vi "Begin.vi"() -> (0 "error out":errorcluster)   [LabVIEW 2013]
doc: "Called before other user functions, this VI is expected to open initial I/O refnums, load in file data, and do all program initialization. Notice that the <B>error out</B> terminal is simply used for data flow. Wiring it to other structures or subVIs ensures that this VI runs first."
uses:
  <vilib>/Rock Robotics/WPI/Camera/WPI_CameraImageSize.ctl
  <vilib>/Rock Robotics/SystemInterfaces/DIO/FPGA_DIOPWMChannel.ctl
  <vilib>/Rock Robotics/WPI/DriverStation/WPI_DriverStationRobotMode2.ctl
  <vilib>/Rock Robotics/WPI/Joystick/WPI_JoystickDeviceEnum.ctl
  <vilib>/Rock Robotics/SystemInterfaces/DIO/FPGA_DIOChannel.ctl
  <vilib>/Rock Robotics/WPI/Encoder/WPI_EncoderType.ctl
  <vilib>/Rock Robotics/WPI/Camera/WPI_CameraWhite Balance Values.ctl
  <vilib>/Rock Robotics/WPI/Camera/WPI_CameraExposure Values.ctl
  <vilib>/Rock Robotics/WPI/Camera/WPI_CameraFrameRate.ctl
  <vilib>/Rock Robotics/WPI/Solenoid/WPI_SolenoidChannel.ctl
  <vilib>/Rock Robotics/SystemInterfaces/DIO/FPGA_DIORelayChannel.ctl
  <vilib>/Rock Robotics/SystemInterfaces/Typedef/FPGA_TypedefDigitalModule.ctl
  <vilib>/Rock Robotics/SystemInterfaces/Typedef/FPGA_TypedefSolenoidModule.ctl
  <vilib>/Rock Robotics/SystemInterfaces/Typedef/FPGA_TypedefAnalogModule.ctl
  <vilib>/Rock Robotics/SystemInterfaces/AI/FPGA_AIChannel.ctl
  <vilib>/Rock Robotics/WPI/Relay/WPI_RelayDirection.ctl
  <vilib>/Rock Robotics/WPI/RobotDrive/WPI_RobotDriveOpen2MotorWithTalon.vi
  Robot Global Data.vi
  <vilib>/Rock Robotics/WPI/MotorControl/WPI_MotorControlOpen Talon.vi
  <vilib>/Rock Robotics/WPI/Counter/WPI_CounterDigitalInputToDigitalSource.vi
  <vilib>/Rock Robotics/WPI/Solenoid/WPI_SolenoidOpenDouble.vi
  <vilib>/Rock Robotics/WPI/Compressor/WPI_CompressorGetSetRefNum.vi
panel:
  in  "Image Size 2":T1=enum."160x120"
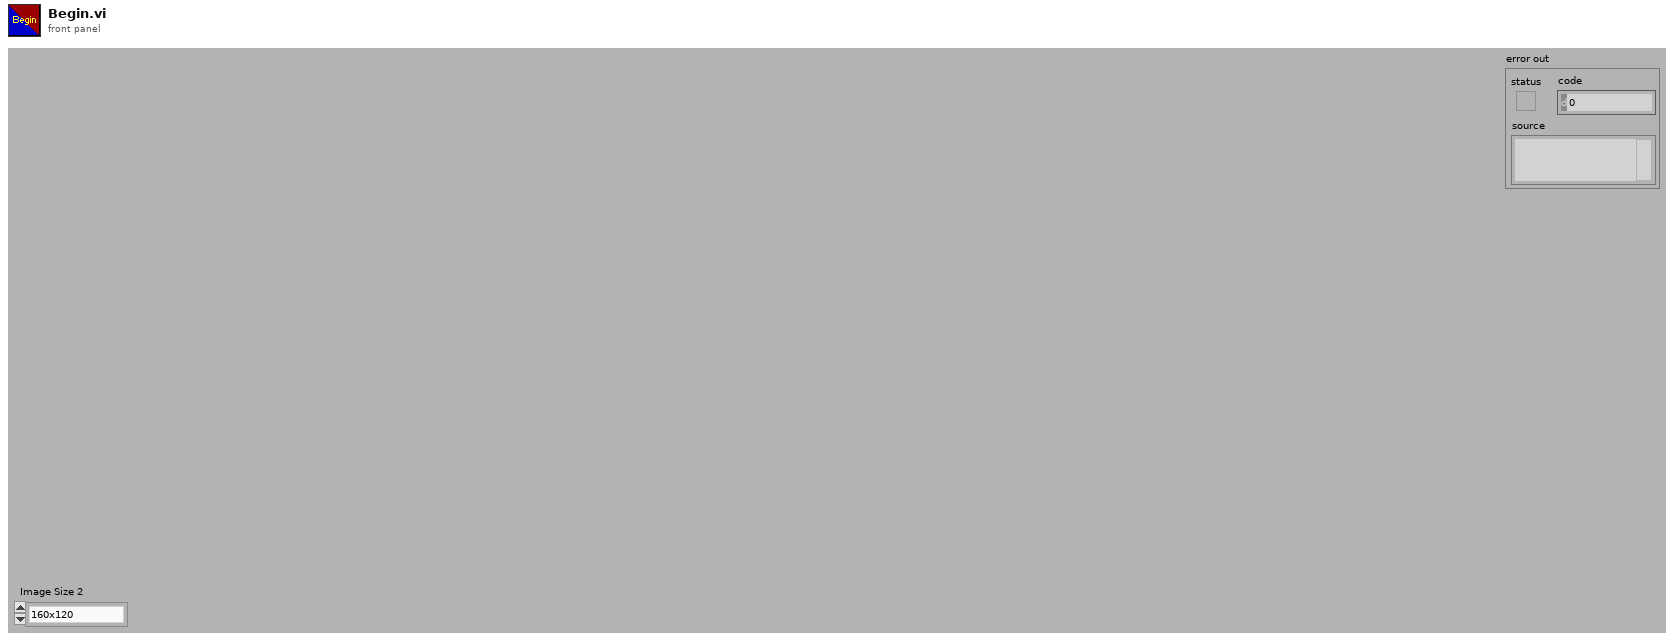
[diagram p1: front panel]
types:
  T1 = typedef "WPI_CameraImageSize.ctl" = enum16{"640x480", "320x240", "160x120"}
  T2 = typedef "WPI_RelayDirection.ctl" = enum16{"Both directions", "Forward only", "Reverse only"}
  T3 = typedef "FPGA_DIORelayChannel.ctl" = enum8{"Relay 1", "Relay 2", "Relay 3", "Relay 4", "Relay 5", "Relay 6", "Relay 7", "Relay 8", "Invalid"}
  T4 = typedef "FPGA_TypedefDigitalModule.ctl" = enum16{"Digital Module 1", "Digital Module 2"}
  T5 = typedef "FPGA_DIOChannel.ctl" = enum8{"DIO 1", "DIO 2", "DIO 3", "DIO 4", "DIO 5", "DIO 6", "DIO 7", "DIO 8", "DIO 9", "DIO 10", "DIO 11", "DIO 12", "DIO 13", "DIO 14", "Invalid"}
  T6 = typedef "WPI_EncoderType.ctl" = enum16{"1x", "2x", "4x"}
  T7 = typedef "FPGA_AIChannel.ctl" = enum8{"AI 1", "AI 2", "AI 3", "AI 4", "AI 5", "AI 6", "AI 7", "AI 8", "Invalid"}
  T8 = typedef "FPGA_TypedefAnalogModule.ctl" = enum16{"Analog Module 1", "Analog Module 2"}
  T9 = typedef "WPI_SolenoidChannel.ctl" = enum8{"Solenoid 1", "Solenoid 2", "Solenoid 3", "Solenoid 4", "Solenoid 5", "Solenoid 6", "Solenoid 7", "Solenoid 8", "Invalid"}
  T10 = typedef "FPGA_TypedefSolenoidModule.ctl" = enum16{"Solenoid Module 1", "Solenoid Module 2"}
  T11 = typedef "FPGA_DIOPWMChannel.ctl" = enum8{"PWM 1", "PWM 2", "PWM 3", "PWM 4", "PWM 5", "PWM 6", "PWM 7", "PWM 8", "PWM 9", "PWM 10", "Invalid"}
  T12 = typedef "WPI_CameraFrameRate.ctl" = u32
  T13 = typedef "WPI_CameraExposure Values.ctl" = enum16{"Auto", "Flicker-free 50 Hz", "Flicker-free 60 Hz", "Hold current"}
  T14 = typedef "WPI_CameraWhite Balance Values.ctl" = enum16{"Auto", "Fixed indoor", "Fixed outdoor 1", "Fixed outdoor 2", "Fixed fluorescent 1", "Fixed fluorescent 2", "Hold current"}
  T15 = typedef "WPI_JoystickDeviceEnum.ctl" = enum16{"USB 1", "USB 2", "USB 3", "USB 4", "Kinect 1", "Kinect 2"}
  T16 = typedef "WPI_DriverStationRobotMode2.ctl" = enum16{"Autonomous Disabled", "Autonomous Enabled", "Teleop Disabled", "Teleop Enabled", "Timeout", "Finish", "Test Disabled", "Test Enabled"}
  T17 = typedef "WPI_JoystickDevRef.ctl" = cluster{"Device":T15}
  T18 = typedef "WPI_DigitalInputDevRef.ctl" = cluster{"DevStatus":errorcluster, "DIO Channel":T5, "Digital Module":T4}
  T19 = typedef "WPI_CompressorDevRef.ctl" = cluster{"DevStatus":errorcluster, "DigitalInputDevRef":T18, "RelayDevRef":T20}
  T20 = typedef "WPI_RelayDevRef.ctl" = cluster{"DevStatus":errorcluster, "Relay Channel":T3, "Digital Module":T4, "Relay Direction":T2}
  T21 = typedef "WPI_RobotDriveDevRef.ctl" = cluster{"DevStatus":errorcluster, "Motors[]":T22[], "Square Inputs":bool, "Max Output":dbl, "Isochronous":bool}
  T22 = typedef "WPI_MotorControlDeviceRef.ctl" = cluster{"DeviceStatus":errorcluster, "Type":enum16{"PWM", "CAN"}, "PWM":cluster{"Digital Module":T4, "PWM Channel":T11, "DeadBand":T23}, "CAN":cluster{"Device Number":u8, "Control Mode":T24, "Semaphore":T25, "Max Vout":dbl}, "Invert":bool, "TransformRef":T26, "InvTransformRef":T26}
  T23 = typedef "WPI_PWMDeadband.ctl" = cluster{"Name":string, "maxPositivePwm":i32, "minPositivePwm":i32, "centerPwm":i32, "maxNegativePwm":i32, "minNegativePwm":i32, "angularRange":u16}
  T24 = typedef "WPI_CANJaguar_ControlMode.ctl" = enum8{"Percent VBus", "Current", "Speed", "Position", "Voltage"}
  T25 = typedef "Semaphore RefNum" = refnum<k1>
  T26 = typedef "WPI_PWMTransform_ConPane.ctl" = refnum<vi>
  T27 = typedef "WPI_SolenoidDevRef.ctl" = cluster{"DevStatus":errorcluster, "Solenoid Module":T10, "Forward Solenoid Channel":T9, "Reverse Solenoid Channel":T9}
  T28 = typedef "FPGA_CounterEncoderSourceConvertionLVSourceType.ctl" = cluster{"DevStatus":errorcluster, "AnalogTriggerMode?":bool, "DigitalMode":cluster{"Digital Module":T4, "DIO Channel":T29}, "AnalogTriggerMode":cluster{"AnalogTriggerIndex":T30, "OutputType":T31}}
  T29 = typedef "FPGA_DIODigitalSourceChannel.ctl" = enum8{"DIO 1", "DIO 2", "DIO 3", "DIO 4", "DIO 5", "DIO 6", "DIO 7", "DIO 8", "DIO 9", "DIO 10", "DIO 11", "DIO 12", "DIO 13", "DIO 14", "Disabled"}
  T30 = typedef "FPGA_AnalogTriggerIndex.ctl" = enum8{"Trig 0", "Trig 1", "Trig 2", "Trig 3", "Trig 4", "Trig 5", "Trig 6", "Trig 7", "Invalid"}
  T31 = typedef "FPGA_AnalogTriggerOutType.ctl" = enum16{"InWindow", "TriggerState", "Rising", "Falling"}
  T32 = typedef "WPI_EncoderDevRef.ctl" = cluster{"DevStatus":errorcluster, "EncoderIndex":T33, "CounterIndex":T34, "DistancePerCount":dbl, "Decoding Type":T6}
  T33 = typedef "FPGA_EncoderIdx.ctl" = enum8{"Enc 0", "Enc 1", "Enc 2", "Enc 3", "Invalid"}
  T34 = typedef "FPGA_CounterCtrSystemIndex.ctl" = enum8{"Ctr 0", "Ctr 1", "Ctr 2", "Ctr 3", "Ctr 4", "Ctr 5", "Ctr 6", "Ctr 7", "Invalid"}
  T35 = typedef "WPI_CameraDevRef.ctl" = cluster{"Camera Address":string, "CameraStatus":errorcluster, "Acquire Image Notifier":refnum<notifier>}
  T36 = typedef "WPI_ServoDeviceRef.ctl" = cluster{"DeviceStatus":errorcluster, "Digital Module":T4, "PWM Channel":T11, "DeadBand":T23}
  T37 = typedef "WPI_AnalogChannelDevRef.ctl" = cluster{"DevStatus":errorcluster, "Analog Module":T8, "Analog Channel":T7}
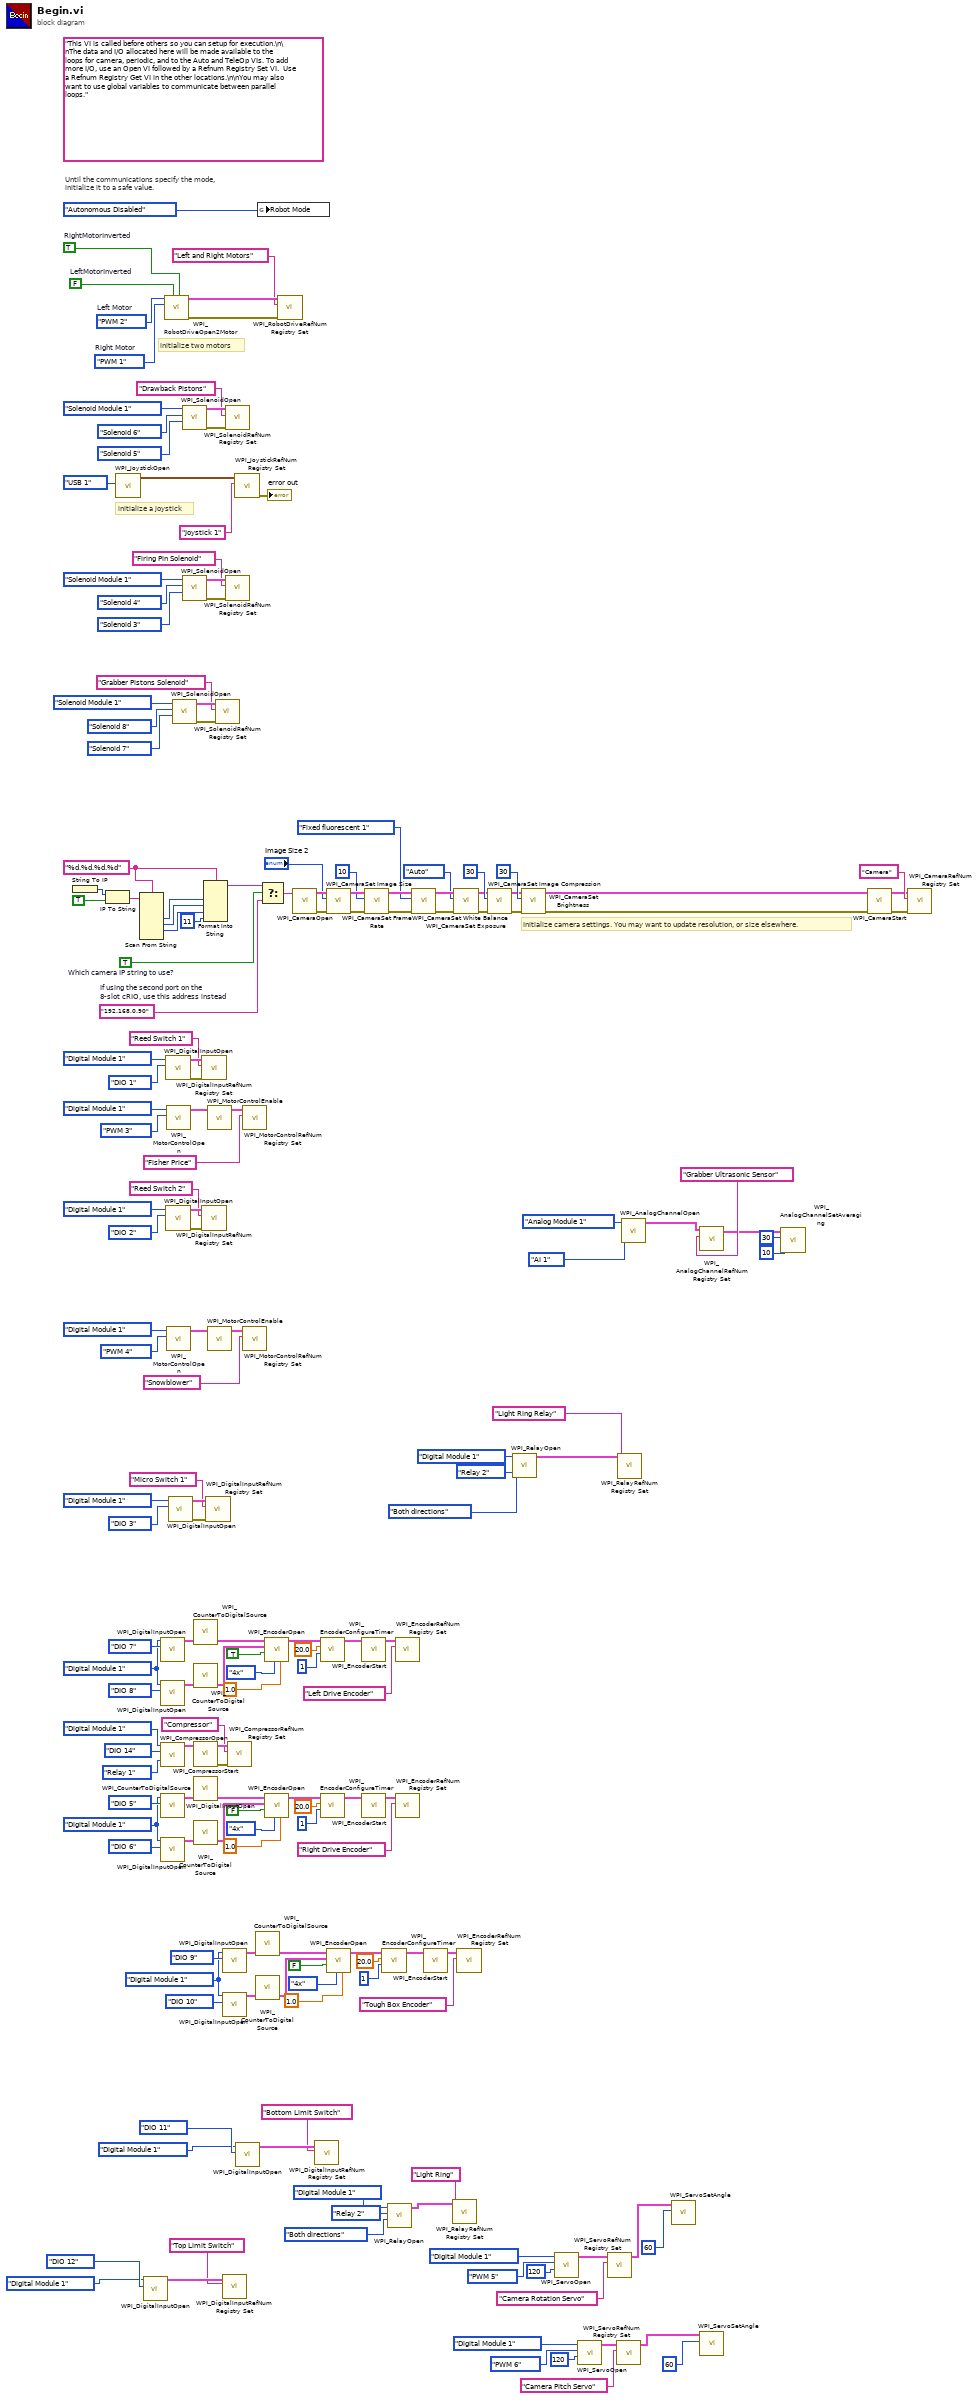
[diagram p0: block diagram]
diagram:
  w22 = FPGA_TypedefDigitalModule."Digital Module 1" ("DIO Module")
  w69 = FPGA_TypedefDigitalModule."Digital Module 1" ("DIO Module")
  w121 = TRUE  # Which camera IP string to use?
  w125 = "%d.%d.%d.%d" ("format string")
  w122 = "192.168.0.90"  # If using the second port on the 8-slot cRIO, use this address instead
  w154 = FPGA_TypedefDigitalModule."Digital Module 1" ("DIO Module")
  (unwired) "This VI is called before others so you can setup for execution.\n\nThe data and I/O allocated here will be made available to the loops for camera, periodic, and to the Auto and TeleOp VIs. To add more I/O, use an Open VI followed by a Refnum Registry Set VI.  Use a Refnum Registry Get VI in the other locations.\n\nYou may also want to use global variables to communicate between parallel loops."
  w178 = FPGA_DIOPWMChannel."PWM 1"  # Right Motor
  w179 = FPGA_DIOPWMChannel."PWM 2"  # Left Motor
  w183 = FALSE  # LeftMotorInverted
  w184 = TRUE  # RightMotorInverted
  # "Initialize camera settings. You may want to update resolution, or size elsewhere."
  # "initialize a joystick"
  # "Until the communications specify the mode,\ninitialize it to a safe value."
  # "initialize two motors"
  n1 = String To IP() -> (0:w132:u32)  [unwired: 1 in]
  n2 = IP To String(1:TRUE ("dot notation? (F)"), 2:w132) -> (0:w130:string)
  n3 = call <vilib>:"WPI_JoystickOpen.vi"("JoystickDevice"=WPI_JoystickDeviceEnum."USB 1") -> ("JoystickDevRef"=w175:T17)  [unwired: 10 in]
  n4 = Scan From String(format string=w125, input string=w130) -> (output 1=w129:i32, output 2=w128:i32, output 3=w127:i32)  [unwired: 7 in, 3 out]
  n5 = call <vilib>:"WPI_DigitalInputOpen.vi"("DIO Channel"=FPGA_DIOChannel."DIO 12" ("A Channel"), "Digital Module (Module 1)"=FPGA_TypedefDigitalModule."Digital Module 1" ("DIO Module")) -> ("DigitalInputDevRef"=w37:T18)  [unwired: 8 in, 1 out]
  n6 = call <vilib>:"WPI_DigitalInputOpen.vi"("DIO Channel"=FPGA_DIOChannel."DIO 7" ("A Channel"), "Digital Module (Module 1)"=w22) -> ("DigitalInputDevRef"=w33:T18)  [unwired: 1 in, 8 out]
  n7 = call <vilib>:"WPI_DigitalInputOpen.vi"("DIO Channel"=FPGA_DIOChannel."DIO 8" ("B Channel"), "Digital Module (Module 1)"=w22) -> ("DigitalInputDevRef"=w34:T18)  [unwired: 1 in, 8 out]
  n8 = call <vilib>:"WPI_CompressorOpen.vi"("Pressure Switch Digital Module (Module 1)"=FPGA_TypedefDigitalModule."Digital Module 1" ("Switch and Relay Module"), "Pressure Switch DIO Channel"=FPGA_DIOChannel."DIO 14" ("Pressure Switch Channel"), "Relay Channel"=FPGA_DIORelayChannel."Relay 1" ("RelayChannel")) -> ("CompressorDevRef"=w109:T19)  [unwired: 2 in, 10 out]
  n9 = call <vilib>:"WPI_DigitalInputOpen.vi"("DIO Channel"=FPGA_DIOChannel."DIO 5" ("A Channel"), "Digital Module (Module 1)"=w154) -> ("DigitalInputDevRef"=w165:T18)  [unwired: 1 in, 8 out]
  n10 = call <vilib>:"WPI_DigitalInputOpen.vi"("DIO Channel"=FPGA_DIOChannel."DIO 6" ("B Channel"), "Digital Module (Module 1)"=w154) -> ("DigitalInputDevRef"=w166:T18)  [unwired: 1 in, 8 out]
  n11 = call-poly <vilib>:"WPI_RobotDriveOpen2Motor.vi"("Right Motor Inverted"=w184, "Left Motor Inverted"=w183, "Right Motor"=w178, "Left Motor"=w179) -> ("error out"=w180:errorcluster, "RobotDriveDevRef"=w182:T21)  [unwired: 1 in, 5 out]
  n12 = call <vilib>:"WPI_DigitalInputOpen.vi"("DIO Channel"=FPGA_DIOChannel."DIO 1" ("Limit Switch Channel"), "Digital Module (Module 1)"=FPGA_TypedefDigitalModule."Digital Module 1" ("Switch and Relay Module")) -> ("error out"=w108:errorcluster, "DigitalInputDevRef"=w107:T18)  [unwired: 1 in, 7 out]
  n13 = call <vilib>:"WPI_DigitalInputOpen.vi"("DIO Channel"=FPGA_DIOChannel."DIO 2" ("Limit Switch Channel"), "Digital Module (Module 1)"=FPGA_TypedefDigitalModule."Digital Module 1" ("Switch and Relay Module")) -> ("error out"=w90:errorcluster, "DigitalInputDevRef"=w89:T18)  [unwired: 1 in, 7 out]
  n14 = call-poly <vilib>:"WPI_MotorControlOpen.vi"("PWM Channel"=FPGA_DIOPWMChannel."PWM 3" ("Left Motor"), "Digital Module (Module 1)"=enum16{"Digital Module 1"}."Digital Module 1") -> ("MotorControlDeviceRef"=w86:T22)  [unwired: 8 in, 1 out]
  n15 = call-poly <vilib>:"WPI_MotorControlOpen.vi"("PWM Channel"=FPGA_DIOPWMChannel."PWM 4" ("Left Motor"), "Digital Module (Module 1)"=enum16{"Digital Module 1"}."Digital Module 1") -> ("MotorControlDeviceRef"=w84:T22)  [unwired: 8 in, 1 out]
  n16 = call <vilib>:"WPI_DigitalInputOpen.vi"("DIO Channel"=FPGA_DIOChannel."DIO 3", "Digital Module (Module 1)"=FPGA_TypedefDigitalModule."Digital Module 1") -> ("error out"=w16:errorcluster, "DigitalInputDevRef"=w17:T18)  [unwired: 1 in, 7 out]
  n17 = call-poly <vilib>:"WPI_SolenoidOpen.vi"("Reverse Solenoid Channel"=WPI_SolenoidChannel."Solenoid 7" ("Extend Solenoid Channel"), "Forward Solenoid Channel"=WPI_SolenoidChannel."Solenoid 8" ("Retract Solenoid Channel"), "Solenoid Module (Module 1)"=FPGA_TypedefSolenoidModule."Solenoid Module 1" ("Solenoid Module")) -> ("error out"=w49:errorcluster, "SolenoidDevRef"=w48:T27)  [unwired: 1 in, 6 out]
  n18 = call-poly <vilib>:"WPI_SolenoidOpen.vi"("Reverse Solenoid Channel"=WPI_SolenoidChannel."Solenoid 5" ("Extend Solenoid Channel"), "Forward Solenoid Channel"=WPI_SolenoidChannel."Solenoid 6" ("Retract Solenoid Channel"), "Solenoid Module (Module 1)"=FPGA_TypedefSolenoidModule."Solenoid Module 1" ("Solenoid Module")) -> ("error out"=w105:errorcluster, "SolenoidDevRef"=w104:T27)  [unwired: 1 in, 6 out]
  n19 = call-poly <vilib>:"WPI_SolenoidOpen.vi"("Reverse Solenoid Channel"=WPI_SolenoidChannel."Solenoid 3" ("Extend Solenoid Channel"), "Forward Solenoid Channel"=WPI_SolenoidChannel."Solenoid 4" ("Retract Solenoid Channel"), "Solenoid Module (Module 1)"=FPGA_TypedefSolenoidModule."Solenoid Module 1" ("Solenoid Module")) -> ("error out"=w96:errorcluster, "SolenoidDevRef"=w95:T27)  [unwired: 1 in, 6 out]
  n20 = call-poly <vilib>:"WPI_CounterToDigitalSource.vi"("DigitalInputDevRef"=w33) -> ("Digital Source"=w32:T28)  [unwired: 6 out]
  n21 = call-poly <vilib>:"WPI_CounterToDigitalSource.vi"("DigitalInputDevRef"=w34) -> ("Digital Source"=w35:T28)  [unwired: 6 out]
  n22 = call <vilib>:"WPI_CompressorStart.vi"("CompressorDevRef"=w109) -> ("error out"=w102:errorcluster, "CompressorDevRef"=w101:T19)  [unwired: 1 in, 8 out]
  n23 = call-poly <vilib>:"WPI_CounterToDigitalSource.vi"("DigitalInputDevRef"=w165) -> ("Digital Source"=w164:T28)  [unwired: 6 out]
  n24 = call-poly <vilib>:"WPI_CounterToDigitalSource.vi"("DigitalInputDevRef"=w166) -> ("Digital Source"=w167:T28)  [unwired: 6 out]
  n25 = call <vilib>:"WPI_DigitalInputRefNum Registry Set.vi"("error in (no error)"=w108, "refnum name"="Reed Switch 1", "DigitalInputDevRef"=w107) -> ()  [unwired: 7 in, 2 out]
  n26 = call <vilib>:"WPI_DigitalInputRefNum Registry Set.vi"("error in (no error)"=w90, "refnum name"="Reed Switch 2", "DigitalInputDevRef"=w89) -> ()  [unwired: 7 in, 2 out]
  n27 = Format Into String(format string=w125, w129, w128, w127, 11 ("Compression")) -> (resulting string=w123:string)  [unwired: 2 in, 1 out]
  n28 = call <vilib>:"WPI_DigitalInputRefNum Registry Set.vi"("error in (no error)"=w16, "refnum name"="Micro Switch 1", "DigitalInputDevRef"=w17) -> ()  [unwired: 7 in, 2 out]
  n29 = call <vilib>:"WPI_MotorControlEnable.vi"("CAN Jaguar Ref"=w86) -> ("CAN Jaguar Ref Out"=w85:T22)  [unwired: 9 in, 1 out]
  n30 = call <vilib>:"WPI_MotorControlEnable.vi"("CAN Jaguar Ref"=w84) -> ("CAN Jaguar Ref Out"=w83:T22)  [unwired: 9 in, 1 out]
  n31 = call <vilib>:"WPI_SolenoidRefNum Registry Set.vi"("error in (no error)"=w49, "refnum name"="Grabber Pistons Solenoid", "SolenoidDevRef"=w48) -> ()  [unwired: 7 in, 2 out]
  n32 = call <vilib>:"WPI_DigitalInputOpen.vi"("DIO Channel"=FPGA_DIOChannel."DIO 9" ("A Channel"), "Digital Module (Module 1)"=w69) -> ("DigitalInputDevRef"=w80:T18)  [unwired: 1 in, 8 out]
  n33 = call <vilib>:"WPI_DigitalInputOpen.vi"("DIO Channel"=FPGA_DIOChannel."DIO 10" ("B Channel"), "Digital Module (Module 1)"=w69) -> ("DigitalInputDevRef"=w81:T18)  [unwired: 1 in, 8 out]
  n34 = call <vilib>:"WPI_DigitalInputRefNum Registry Set.vi"("refnum name"="Top Limit Switch", "DigitalInputDevRef"=w37) -> ()  [unwired: 8 in, 2 out]
  n35 = call <vilib>:"WPI_SolenoidRefNum Registry Set.vi"("error in (no error)"=w105, "refnum name"="Drawback Pistons", "SolenoidDevRef"=w104) -> ()  [unwired: 7 in, 2 out]
  n36 = call <vilib>:"WPI_SolenoidRefNum Registry Set.vi"("error in (no error)"=w96, "refnum name"="Firing Pin Solenoid", "SolenoidDevRef"=w95) -> ()  [unwired: 7 in, 2 out]
  n37 = call <vilib>:"WPI_CompressorRefNum Registry Set.vi"("error in (no error)"=w102, "refnum name"="Compressor", "CompressorDevRef"=w101) -> ()  [unwired: 7 in, 2 out]
  n38 = call <vilib>:"WPI_JoystickRefNum Registry Set.vi"("refnum name"="Joystick 1", "JoystickDevRef"=w175) -> ("error out"=→"error out":errorcluster)  [unwired: 8 in, 1 out]
  n39 = call <vilib>:"WPI_DigitalInputOpen.vi"("DIO Channel"=FPGA_DIOChannel."DIO 11" ("A Channel"), "Digital Module (Module 1)"=FPGA_TypedefDigitalModule."Digital Module 1" ("DIO Module")) -> ("DigitalInputDevRef"=w64:T18)  [unwired: 8 in, 1 out]
  n40 = call <vilib>:"WPI_MotorControlRefNum Registry Set.vi"("refnum name"="Fisher Price", "MotorControlDevRef"=w85) -> ()  [unwired: 8 in, 2 out]
  n41 = call <vilib>:"WPI_MotorControlRefNum Registry Set.vi"("refnum name"="Snowblower", "MotorControlDevRef"=w83) -> ()  [unwired: 8 in, 2 out]
  n42 = call-poly <vilib>:"WPI_CounterToDigitalSource.vi"("DigitalInputDevRef"=w80) -> ("Digital Source"=w79:T28)  [unwired: 6 out]
  n43 = call-poly <vilib>:"WPI_CounterToDigitalSource.vi"("DigitalInputDevRef"=w81) -> ("Digital Source"=w82:T28)  [unwired: 6 out]
  n44 = global write "Robot Global Data.vi" "Robot Mode"(WPI_DriverStationRobotMode2."Autonomous Disabled" ("Robot Mode")) -> ()
  n45 = Select(t=w123, s=w121, f=w122) -> (s? t:f=w124:string)
  n46 = call <vilib>:"WPI_EncoderOpen.vi"("DistancePerCount"=1.0, "Decoding Type"=WPI_EncoderType."4x", "Invert Direction (False)"=TRUE ("Invert Direction"), "BSource"=w35, "ASource"=w32) -> ("EncoderDevRef"=w25:T32)  [unwired: 3 in, 3 out]
  n47 = call <vilib>:"WPI_EncoderOpen.vi"("DistancePerCount"=1.0, "Decoding Type"=WPI_EncoderType."4x", "Invert Direction (False)"=FALSE ("Invert Direction"), "BSource"=w167, "ASource"=w164) -> ("EncoderDevRef"=w157:T32)  [unwired: 3 in, 3 out]
  n48 = call <vilib>:"WPI_RobotDriveRefNum Registry Set.vi"("error in (no error)"=w180, "refnum name"="Left and Right Motors", "RobotDriveDevRef"=w182) -> ()  [unwired: 9 out]
  n49 = call <vilib>:"WPI_CameraOpen.vi"("Camera Address"=w124) -> ("error out"=w142:errorcluster, "CameraDevRef"=w143:T35)  [unwired: 1 in, 8 out]
  n50 = call <vilib>:"WPI_DigitalInputRefNum Registry Set.vi"("refnum name"="Bottom Limit Switch", "DigitalInputDevRef"=w64) -> ()  [unwired: 8 in, 2 out]
  n51 = call <vilib>:"WPI_EncoderConfigureTimer.vi"("Number Samples to Average"=u8 1, "Minimum Rate"=20.0, "EncoderDevRef"=w25) -> ("EncoderDevRef"=w26:T32)  [unwired: 1 in, 7 out]
  n52 = call <vilib>:"WPI_EncoderConfigureTimer.vi"("Number Samples to Average"=u8 1, "Minimum Rate"=20.0, "EncoderDevRef"=w157) -> ("EncoderDevRef"=w158:T32)  [unwired: 1 in, 7 out]
  n53 = call <vilib>:"WPI_CameraSet Image Size.vi"("error in (no error)"=w142, "Image Size"="Image Size 2", "CameraDevRef"=w143) -> ("error out"=w141:errorcluster, "CameraDevRef Out"=w144:T35)  [unwired: 7 out]
  n54 = call <vilib>:"WPI_EncoderOpen.vi"("DistancePerCount"=1.0, "Decoding Type"=WPI_EncoderType."4x", "Invert Direction (False)"=FALSE ("Invert Direction"), "BSource"=w82, "ASource"=w79) -> ("EncoderDevRef"=w72:T32)  [unwired: 3 in, 3 out]
  n55 = call <vilib>:"WPI_EncoderStart.vi"("EncoderDevRef"=w26) -> ("EncoderDevRef"=w21:T32)  [unwired: 1 in, 9 out]
  n56 = call <vilib>:"WPI_EncoderStart.vi"("EncoderDevRef"=w158) -> ("EncoderDevRef"=w153:T32)  [unwired: 1 in, 9 out]
  n57 = call <vilib>:"WPI_CameraSet Frame Rate.vi"("error in (no error)"=w141, "Frame Rate (fps)"=T12 10, "CameraDevRef"=w144) -> ("error out"=w140:errorcluster, "CameraDevRef Out"=w146:T35)  [unwired: 7 out]
  n58 = call <vilib>:"WPI_EncoderConfigureTimer.vi"("Number Samples to Average"=u8 1, "Minimum Rate"=20.0, "EncoderDevRef"=w72) -> ("EncoderDevRef"=w73:T32)  [unwired: 1 in, 7 out]
  n59 = call <vilib>:"WPI_RelayOpen.vi"("Relay Direction"=WPI_RelayDirection."Both directions", "Relay Channel"=FPGA_DIORelayChannel."Relay 2", "Digital Module (Module 1)"=FPGA_TypedefDigitalModule."Digital Module 1") -> ("RelayDevRef"=w6:T20)  [unwired: 7 in, 1 out]
  n60 = call <vilib>:"WPI_EncoderRefNum Registry Set.vi"("refnum name"="Left Drive Encoder", "EncoderDevRef"=w21) -> ()  [unwired: 8 in, 2 out]
  n61 = call <vilib>:"WPI_EncoderRefNum Registry Set.vi"("refnum name"="Right Drive Encoder", "EncoderDevRef"=w153) -> ()  [unwired: 8 in, 2 out]
  n62 = call <vilib>:"WPI_CameraSet White Balance.vi"("error in (no error)"=w140, "White Balance"=WPI_CameraWhite_Balance_Values."Fixed fluorescent 1", "CameraDevRef"=w146) -> ("error out"=w139:errorcluster, "CameraDevRef Out"=w145:T35)  [unwired: 7 out]
  n63 = call <vilib>:"WPI_EncoderStart.vi"("EncoderDevRef"=w73) -> ("EncoderDevRef"=w68:T32)  [unwired: 1 in, 9 out]
  n64 = call <vilib>:"WPI_RelayRefNum Registry Set.vi"("refnum name"="Light Ring", "RelayDevRef"=w6) -> ()  [unwired: 8 in, 2 out]
  n65 = call <vilib>:"WPI_CameraSet Exposure.vi"("error in (no error)"=w139, "Exposure"=WPI_CameraExposure_Values."Auto", "CameraDevRef"=w145) -> ("error out"=w138:errorcluster, "CameraDevRef Out"=w148:T35)  [unwired: 7 out]
  n66 = call <vilib>:"WPI_EncoderRefNum Registry Set.vi"("refnum name"="Tough Box Encoder", "EncoderDevRef"=w68) -> ()  [unwired: 8 in, 2 out]
  n67 = call <vilib>:"WPI_CameraSet Image Compression.vi"("error in (no error)"=w138, "Compression"=30, "CameraDevRef"=w148) -> ("error out"=w137:errorcluster, "CameraDevRef Out"=w147:T35)  [unwired: 7 out]
  n68 = call <vilib>:"WPI_RelayOpen.vi"("Relay Direction"=WPI_RelayDirection."Both directions", "Relay Channel"=FPGA_DIORelayChannel."Relay 2", "Digital Module (Module 1)"=FPGA_TypedefDigitalModule."Digital Module 1") -> ("RelayDevRef"=w11:T20)  [unwired: 7 in, 1 out]
  n69 = call <vilib>:"WPI_CameraSet Brightness.vi"("error in (no error)"=w137, "Brightness"=30, "CameraDevRef"=w147) -> ("error out"=w120:errorcluster, "CameraDevRef Out"=w119:T35)  [unwired: 7 out]
  n70 = call <vilib>:"WPI_ServoOpen.vi"("Angular Range"=u16 120, "PWM Channel"=FPGA_DIOPWMChannel."PWM 5", "Digital Module (Module 1)"=FPGA_TypedefDigitalModule."Digital Module 1") -> ("ServoDeviceRef"=w55:T36)  [unwired: 7 in, 1 out]
  n71 = call <vilib>:"WPI_ServoOpen.vi"("Angular Range"=u16 120, "PWM Channel"=FPGA_DIOPWMChannel."PWM 6", "Digital Module (Module 1)"=FPGA_TypedefDigitalModule."Digital Module 1") -> ("ServoDeviceRef"=w56:T36)  [unwired: 7 in, 1 out]
  n72 = call <vilib>:"WPI_ServoRefNum Registry Set.vi"("refnum name"="Camera Rotation Servo", "ServoDeviceRef"=w55) -> ("ServoDeviceRef"=w4:T36)  [unwired: 8 in, 1 out]
  n73 = call <vilib>:"WPI_ServoRefNum Registry Set.vi"("refnum name"="Camera Pitch Servo", "ServoDeviceRef"=w56) -> ("ServoDeviceRef"=w2:T36)  [unwired: 8 in, 1 out]
  n74 = call <vilib>:"WPI_RelayRefNum Registry Set.vi"("refnum name"="Light Ring Relay", "RelayDevRef"=w11) -> ()  [unwired: 8 in, 2 out]
  n75 = call <vilib>:"WPI_AnalogChannelOpen.vi"("Analog Channel"=FPGA_AIChannel."AI 1", "Analog Module (Module 1)"=FPGA_TypedefAnalogModule."Analog Module 1") -> ("AIDeviceRef"=w44:T37)  [unwired: 8 in, 1 out]
  n76 = call <vilib>:"WPI_ServoSetAngle.vi"("Angle"=60, "ServoDeviceRef"=w4) -> ()  [unwired: 8 in, 2 out]
  n77 = call <vilib>:"WPI_AnalogChannelRefNum Registry Set.vi"("refnum name"="Grabber Ultrasonic Sensor", "AIDeviceRef"=w44) -> ("AIDeviceRef"=w42:T37)  [unwired: 8 in, 1 out]
  n78 = call <vilib>:"WPI_ServoSetAngle.vi"("Angle"=60, "ServoDeviceRef"=w2) -> ()  [unwired: 8 in, 2 out]
  n79 = call <vilib>:"WPI_AnalogChannelSetAveraging.vi"("OversampleBits"=u8 10, "AverageBits"=u8 30, "AIDeviceRef"=w42) -> ()  [unwired: 7 in, 2 out]
  n80 = call <vilib>:"WPI_CameraStart.vi"("error in (no error)"=w120, "CameraDevRef"=w119) -> ("error out"=w118:errorcluster, "CameraDevRef Out"=w117:T35)  [unwired: 8 in]
  n81 = call <vilib>:"WPI_CameraRefNum Registry Set.vi"("error in (no error)"=w118, "refnum name"="Camera", "CameraDevRef"=w117) -> ()  [unwired: 9 out]
